vi "VariantToDescriptorElements.vi"(10 "Variant":variant) -> (1 "name":string, 2 "Descriptors":T1[](array[typedef]))   [LabVIEW 2013, in "OpenDescriptor.lvlib"]
uses:
  OpenDescriptor.lvlib
  OpenDescriptor -- cluster.ctl
  TypeDescriptor_GetPString.vi
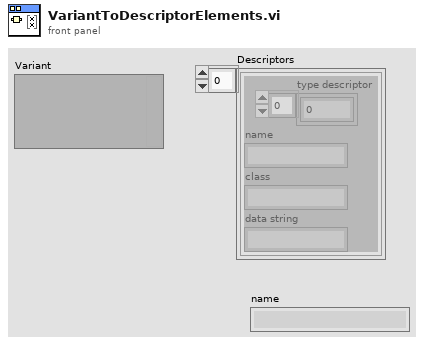
[diagram p1: front panel]
types:
  T1 = typedef "OpenDescriptor.lvlib/OpenDescriptor -- cluster.ctl" = cluster{"type descriptor":i16[], "name":string, "class":string, "data string":string}
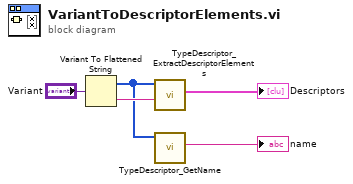
[diagram p0: block diagram]
diagram:
  n1 = Variant To Flattened String(Variant="Variant") -> (data string=w4:string, 1:w2:i16[])
  n2 = call "TypeDescriptor_ExtractDescriptorElements.vi"("Data String"=w4, "type descriptor"=w2) -> ("elements"=→"Descriptors":T1[])  [unwired: 6 in, 3 out]
  n3 = call "TypeDescriptor_GetName.vi"("type descriptor"=w2) -> ("name"=→"name":string)  [unwired: 8 in, 2 out]
